vi "dosimat_wait_till_ready.vi"(2 "error in":errorcluster, 3 "Dosimat Port In":refnum<visa-resource-name>="COM1") -> (0 "error out":errorcluster, 1 "Dosimat Port Out":refnum<visa-resource-name>="COM1")   [LabVIEW 2010]
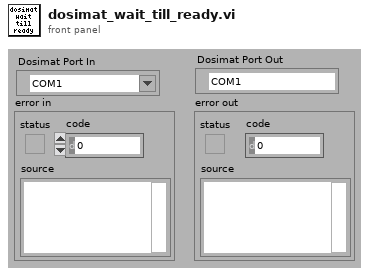
[diagram p1: front panel]
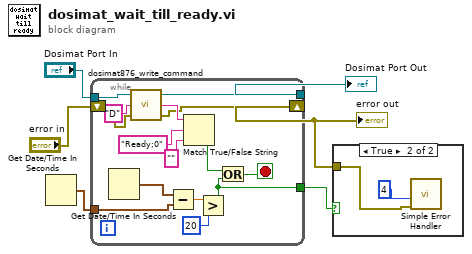
[diagram p0: block diagram]
diagram:
  n1 = Get Date/Time In Seconds() -> (seconds since 1Jan1904=w3:timestamp)
  n2 = while {
    tunnel: "Dosimat Port In" -> [w17]
    tunnel: [w15] -> w4
    shift-right: [w14] -> w1
    shift-left: "error in" -> [w16]
    tunnel: w3 -> [w10]
    tunnel: [w7] -> w2
    stop <- w12 stop-if-true
    n3 = Get Date/Time In Seconds() -> (seconds since 1Jan1904=w9:timestamp)
    n4 = call "dosimat876_write_command.vi"("error in"=w16, "write buffer"="D", "Dosimat Port In"=w17) -> ("error out"=w14:errorcluster, "read buffer"=w18:string, "Dosimat Port Out"=w15:refnum<visa-resource-name>)
    n5 = Subtract(x=w9, y=w10) -> (x-y=w11:dbl)
    n6 = Match True/False String(2:"" ("false string"), 3:"Ready;0" ("true string"), 4:w18) -> (0:w13:bool)  [unwired: 1 out]
    n7 = Greater?(x=w11, y=20) -> (0:w7:bool)
    n8 = Or(x=w13, y=w7) -> (x .or. y?=w12:bool)
  }
  "error out" <- w1
  "Dosimat Port Out" <- w4
  n9 = case shown="True" w2 {
    tunnel: w1 -> [_ w23]
    frame False {
    }
    frame True {
      n10 = call <vilib>:"Simple Error Handler.vi"("type of dialog (OK msg:1)"=4, "error in (no error)"=w23) -> ()  [unwired: 3 in, 5 out]
    }
  }
